vi "Module Init.vi"(8 "error in (no error)":errorcluster, 11 "Messaging Client in":refnum<class "Messaging Server Client.lvclass">) -> (0 "error out":errorcluster, 3 "Messaging Client out":refnum<class "Messaging Server Client.lvclass">)   [LabVIEW 2020, in "Volatus.lvlib" / "Messaging Server Client.lvclass"]
uses:
  Messaging Server Client.lvclass
  Messaging Server Client.lvclass/Messaging Server Client.ctl
  Module/Module.lvclass
  C:/dev/lv20CE/relink/lv-volatus/Volatus/Module/Module.lvclass
  C:/dev/lv20CE/relink/lv-volatus/Volatus/Messaging Client/Messaging Server Client.lvclass
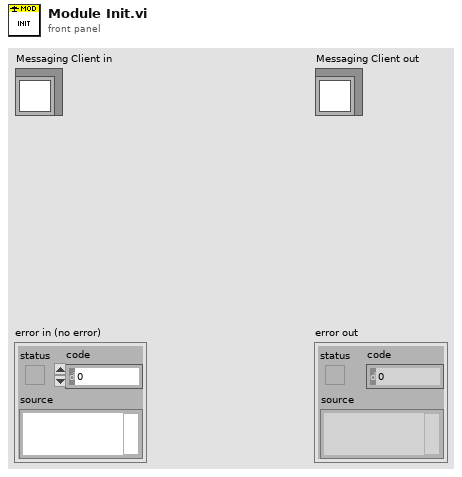
[diagram p1: front panel]
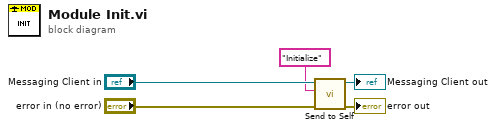
[diagram p0: block diagram]
diagram:
  n1 = call "Send to Self.vi"("error in (no error)"="error in (no error)", "Message ID"="Initialize", "Module in"="Messaging Client in") -> ("error out"=→"error out":errorcluster, "Module out"=→"Messaging Client out":refnum<class "Messaging Server Client.lvclass">)  [unwired: 7 in]
